vi "Utility Filter Out Indicators.vi"(1 "Controls In":refnum<vi>[](array[refnum])) -> (0 "Controls Out":refnum<vi>[](array[refnum]))   [LabVIEW 2020]
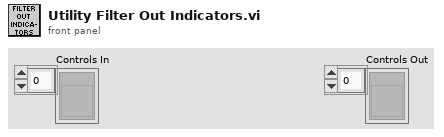
[diagram p1: front panel]
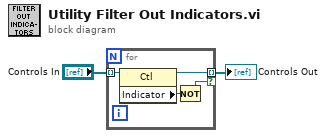
[diagram p0: block diagram]
diagram:
  n1 = for {
    tunnel: "Controls In" -> [w6] mode=indexing
    tunnel: [w5] -> w1 mode=indexing if=w3
    n2 = property class="Ctl"(reference=w6) -> (reference out=w5:refnum<vi>, "Indicator"=w4:bool)  [unwired: 1 in, 1 out]
    n3 = Not(x=w4) -> (.not. x?=w3:bool)
  }
  "Controls Out" <- w1
